vi "ShowCards(Cover).vi"(1 "Array":i16[](array[numeric])) -> (0 "Array 2":u16[](array[ring]))   [LabVIEW 2018]
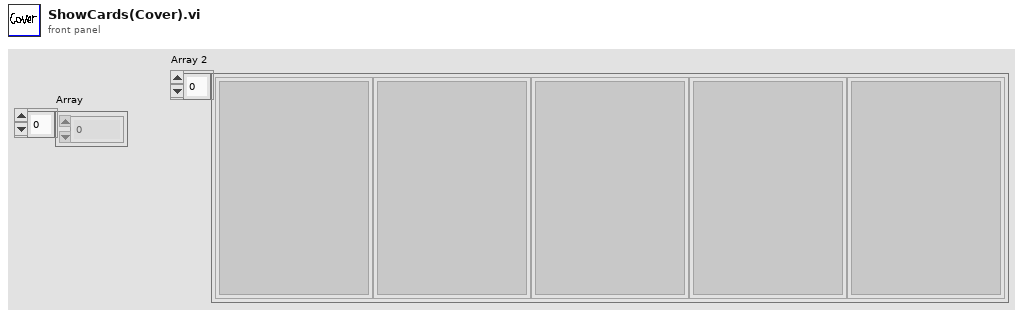
[diagram p1: front panel]
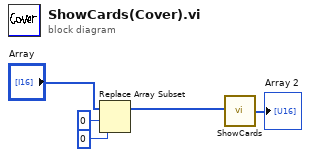
[diagram p0: block diagram]
diagram:
  n1 = Replace Array Subset(array="Array", new element=i16 0 ("新元素/子数组"), index=0 ("索引")) -> (w2:i16[])
  n2 = call "ShowCards.vi"("Array 2"=w2) -> ("Array"=→"Array 2":u16[])
